vi "VISA_Open.vi"() -> ()   [LabVIEW 2020]
panel:
  in  "错误输入":errorcluster caption="错误输入（无错误）"
  in  "VISA资源名称":refnum<visa-resource-name>
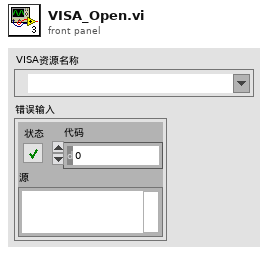
[diagram p1: front panel]
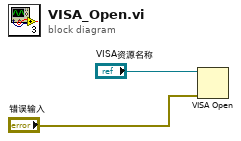
[diagram p0: block diagram]
diagram:
  n1 = VISA Open(error in (no error)="错误输入", VISA resource name="VISA资源名称") -> ()  [unwired: 3 in, 2 out]
